vi "half data samping(50ms).vi"() -> ()   [LabVIEW 2015]
panel:
  out "파일 이름":string[](array[string])
  out "ing":path
  in  "경로":path
  in  "Number of Remove data":i32=4
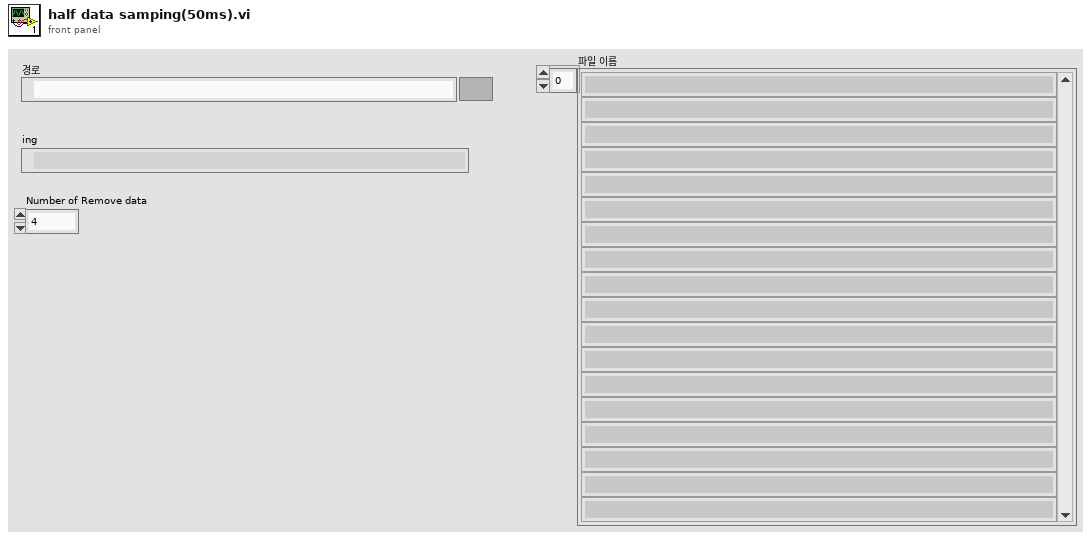
[diagram p1: front panel]
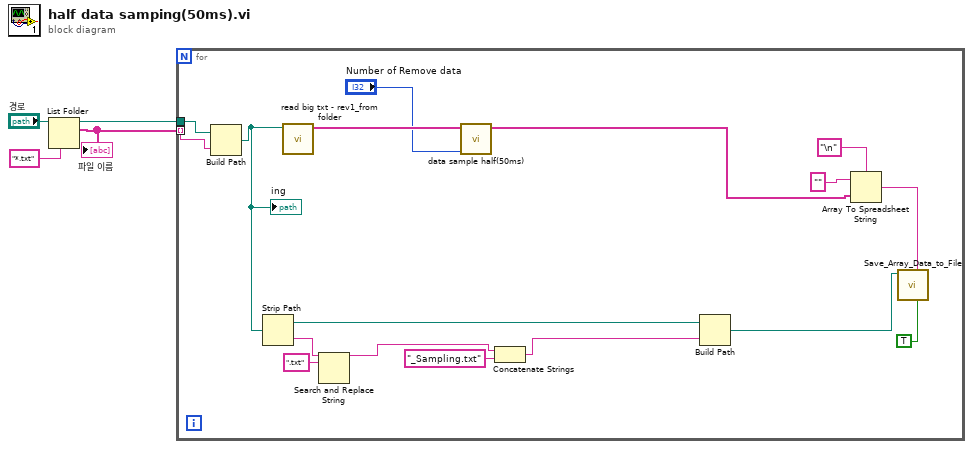
[diagram p0: block diagram]
diagram:
  n1 = List Folder(path="경로", pattern="*.txt" ("패턴")) -> (path out=w3:path, filenames=w2:string[])  [unwired: 2 in, 2 out]
  "파일 이름" <- w2
  n2 = for {
    tunnel: w3 -> [w10]
    tunnel: w2 -> [w9] mode=indexing
    n3 = Build Path(base path=w10, name or relative path=w9) -> (appended path=w8:path)
    "ing" <- w8
    n4 = Strip Path(path=w8) -> (stripped path=w18:path, name=w7:string)
    n5 = call "read big txt - rev1_from folder.vi"("파일 경로(대화 상자 사용)"=w8) -> ("배열"=w14:string[])  [unwired: 10 in]
    n6 = Search and Replace String(input string=w7, search string=".txt" ("검색 문자열")) -> (result string=w5:string)  [unwired: 6 in, 3 out]
    n7 = call "data sample half(50ms).vi"("Number of Remove data"="Number of Remove data", "배열"=w14) -> ("배열 2"=w12:string[])  [unwired: 9 in]
    n8 = Concatenate Strings(w5, "_Sampling.txt" ("문자열")) -> (w16:string)
    n9 = Build Path(base path=w18, name or relative path=w16) -> (appended path=w15:path)
    n10 = Array To Spreadsheet String(delimiter (Tab)="\n" ("구분 문자(탭)"), array=w12, 3:"" ("포맷 문자열")) -> (spreadsheet string=w13:string)
    n11 = call "Save_Array_Data_to_File.vi"("Raw Stiring?"=TRUE, "Raw String"=w13, "file path (use dialog)"=w15) -> ()  [unwired: 8 in, 1 out]
  }
